vi "Clear Pins SubVI.vi"(11 "Pins In":refnum<k21>[](array[refnum])) -> (3 "Pins Out":refnum<k21>[](array[refnum]))   [LabVIEW 2020]
uses:
  <vilib>/DAQmx/write.llb/DAQmx Write (Digital Bool 1Line 1Point).vi
  <vilib>/DAQmx/miscellaneous.llb/DAQmx Fill In Error Info.vi
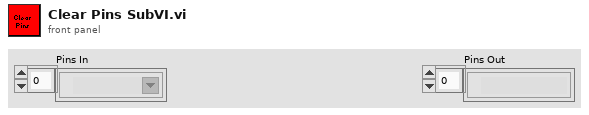
[diagram p1: front panel]
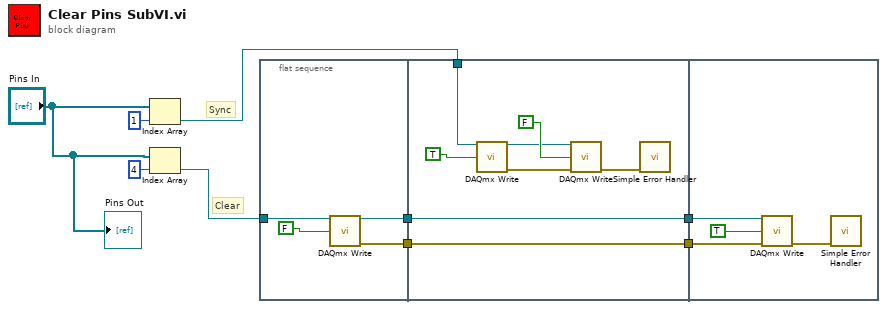
[diagram p0: block diagram]
diagram:
  # "Clear"
  # "Sync"
  n1 = Index Array(array="Pins In", index=1) -> (element=w2:refnum<k21>)
  n2 = Index Array(array="Pins In", index=4) -> (element=w3:refnum<k21>)
  n3 = flat-sequence {
    tunnel: w3 -> [w10]
    tunnel: [w12] -> w9
    tunnel: [w11] -> w7
    tunnel: w9 -> [w16]
    tunnel: [w16] -> w8
    tunnel: w7 -> [w15]
    tunnel: [w15] -> w6
    tunnel: w2 -> [w14]
    tunnel: w8 -> [w22]
    tunnel: w6 -> [w23]
    frame #0 {
      n4 = call-poly <vilib>:"DAQmx Write.vi"("task/channels in"=w10, "data"=FALSE) -> ("task out"=w11:refnum<k21>, "error out"=w12:errorcluster)  [unwired: 11 in, 1 out]
    }
    frame #1 {
      n5 = call-poly <vilib>:"DAQmx Write.vi"("task/channels in"=w14, "data"=TRUE) -> ("task out"=w17:refnum<k21>, "error out"=w18:errorcluster)  [unwired: 11 in, 1 out]
      n6 = call-poly <vilib>:"DAQmx Write.vi"("task/channels in"=w17, "data"=FALSE, "error in"=w18) -> ("error out"=w19:errorcluster)  [unwired: 10 in, 2 out]
      n7 = call <vilib>:"Simple Error Handler.vi"("error in (no error)"=w19) -> ()  [unwired: 4 in, 5 out]
    }
    frame #2 {
      n8 = call-poly <vilib>:"DAQmx Write.vi"("task/channels in"=w23, "data"=TRUE, "error in"=w22) -> ("error out"=w24:errorcluster)  [unwired: 10 in, 2 out]
      n9 = call <vilib>:"Simple Error Handler.vi"("error in (no error)"=w24) -> ()  [unwired: 4 in, 5 out]
    }
  }
  "Pins Out" <- "Pins In"
